vi "Expand FIFO Flags.vi"(11 "FIFO Flags":u64) -> (3 "Flags":T1)   [LabVIEW 2021, in "ChannelCommon.lvlib"]
uses:
  ChannelCommon.lvlib
  typedef/FIFO Flags.ctl
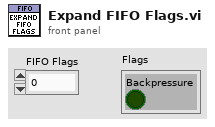
[diagram p1: front panel]
types:
  T1 = typedef "ChannelCommon.lvlib/FIFO Flags.ctl" = cluster{"Backpressure":bool}
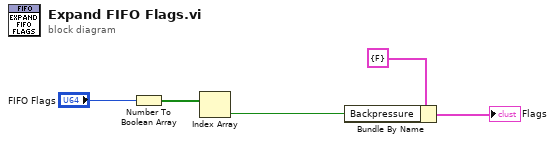
[diagram p0: block diagram]
diagram:
  n1 = Number To Boolean Array(number="FIFO Flags") -> (Boolean array=w4:bool[])
  n2 = Index Array(array=w4) -> (element=w2:bool)  [unwired: 1 in]
  n3 = Bundle By Name(cluster=T1 {"Backpressure"=FALSE} ("Flags"), "Backpressure"=w2) -> (→"Flags":T1)
